vi "Test JSON to Variant (attributes and waveforms).vi"() -> ()   [LabVIEW 2011]
uses:
  JSON Value/Set from JSON string.vi
  JSON Value/Get as JSON string (pretty).vi
  JSON Value/JSON Value.lvclass
  Variant JSON.lvlib
  Get Polymorphic/JSON GetSet.lvlib
panel:
  out "data":T1
  out "Variant out 2":variant
  in  "Attributes cluster":cluster{"T2":string, "Boolean 1":bool, "T1":dbl}={"T2"="Test \"quote\",\nand newline.", "Boolean 1"=TRUE, "T1"=456.789}
  out "JSON String created":string
  # "see diagram"
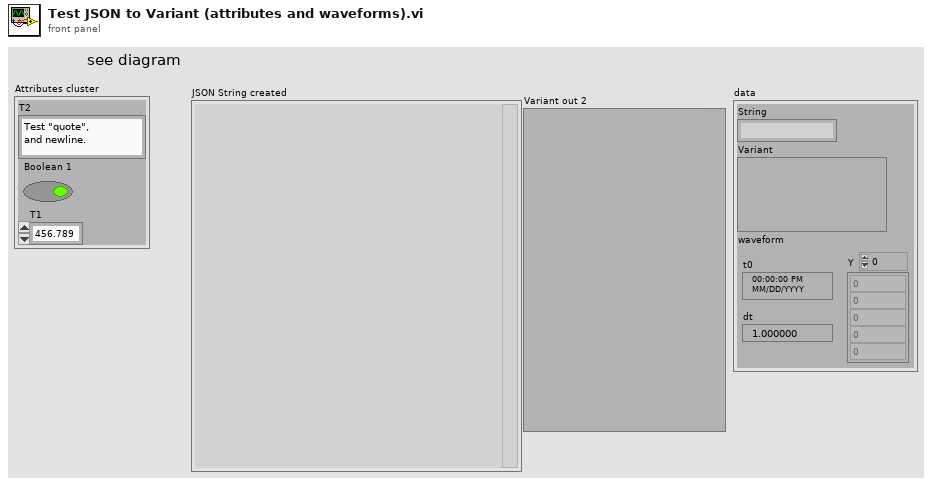
[diagram p1: front panel]
types:
  T1 = cluster{"String":string, "Variant":variant, "waveform":waveform(dbl)}
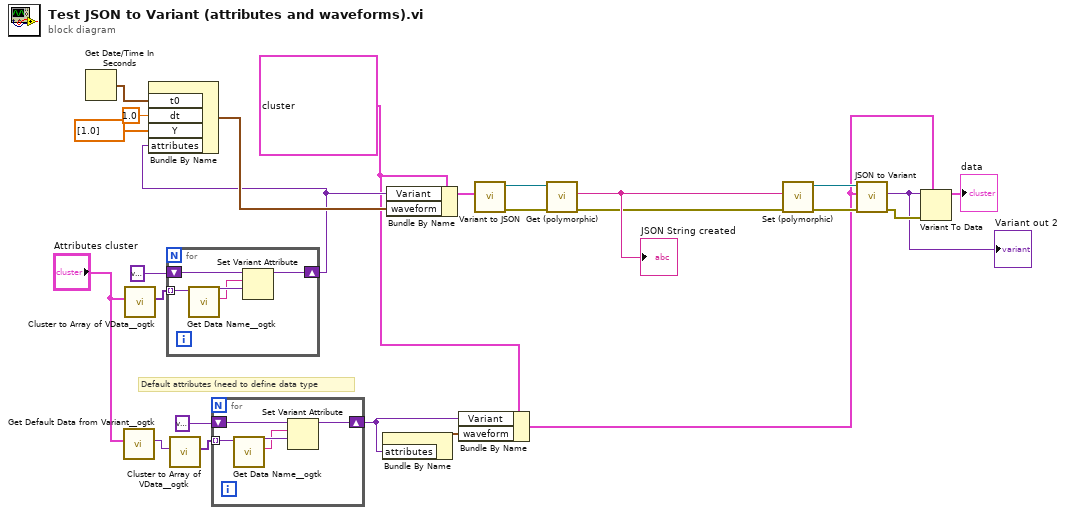
[diagram p0: block diagram]
diagram:
  w4 = T1 {"String"="Test Variant in cluster", "Variant"=variant, "waveform"={"t0"=timestamp(0 s since 1904-01-01), "dt"=1.0, "Y"=[]}}
  # "Default attributes (need to define data type"
  n1 = Get Date/Time In Seconds() -> (seconds since 1Jan1904=w13:timestamp)
  n2 = call <userlib>:"Get Default Data from Variant__ogtk.vi"("Variant"="Attributes cluster") -> ("Default VData"=w5:variant)  [unwired: 9 in, 1 out]
  n3 = call <userlib>:"Cluster to Array of VData__ogtk.vi"("Cluster"="Attributes cluster") -> ("Array of VData"=w20:variant[])  [unwired: 9 in, 1 out]
  n4 = for {
    tunnel: w20 -> [w30] mode=indexing
    shift-right: [w28] -> w9
    shift-left: variant ("Variant") -> [w29]
    n5 = call <userlib>:"Get Data Name__ogtk.vi"("Data"=w30) -> ("Data Name"=w26:string, "Data dup"=w27:variant)  [unwired: 8 in, 1 out]
    n6 = Set Variant Attribute(Variant=w29, name=w26, value=w27) -> (Variant out=w28:variant)  [unwired: 1 in, 2 out]
  }
  n7 = Bundle By Name("t0"=w13, "dt"=1.0, "Y"=dbl[] [1.0], "attributes"=w9) -> (w11:waveform(dbl))  [unwired: 1 in]
  n8 = call <userlib>:"Cluster to Array of VData__ogtk.vi"("Cluster"=w5) -> ("Array of VData"=w6:variant[])  [unwired: 9 in, 1 out]
  n9 = for {
    tunnel: w6 -> [w35] mode=indexing
    shift-right: [w33] -> w3
    shift-left: variant ("Variant") -> [w34]
    n10 = call <userlib>:"Get Data Name__ogtk.vi"("Data"=w35) -> ("Data Name"=w31:string, "Data dup"=w32:variant)  [unwired: 8 in, 1 out]
    n11 = Set Variant Attribute(Variant=w34, name=w31, value=w32) -> (Variant out=w33:variant)  [unwired: 1 in, 2 out]
  }
  n12 = Bundle By Name("attributes"=w3) -> (w1:waveform(dbl))  [unwired: 1 in]
  n13 = Bundle By Name(cluster=w4, "Variant"=w9, "waveform"=w11) -> (w15:T1)
  n14 = Bundle By Name(cluster=w4, "Variant"=w3, "waveform"=w1) -> (w2:T1)
  n15 = call "Variant to JSON.vi"("Variant"=w15) -> ("error out"=w22:errorcluster, "JSON Value out"=w25:refnum<class "JSON Value.lvclass">)  [unwired: 9 in]
  n16 = call-poly "Get (polymorphic).vi"("error in (no error)"=w22, "JSON Value in"=w25) -> ("error out"=w21:errorcluster, "String"=w23:string)  [unwired: 8 in]
  "JSON String created" <- w23
  n17 = call-poly "Set (polymorphic).vi"("error in (no error)"=w21, "JSON stream"=w23) -> ("error out"=w18:errorcluster, "JSON Value out"=w16:refnum<class "JSON Value.lvclass">)  [unwired: 7 in, 1 out]
  n18 = call "JSON to Variant.vi"("error in (no error)"=w18, "Variant (Data Type)"=w2, "JSON Value"=w16) -> ("error out"=w24:errorcluster, "Variant out"=w17:variant)  [unwired: 7 in]
  "Variant out 2" <- w17
  n19 = Variant To Data(error in=w24, type=w2, Variant=w17) -> (data=→"data":T1)  [unwired: 1 out]
